vi "Read Variable (integer).vi"(8 "error in (no error)":errorcluster, 9 "Datatype":i32, 10 "PG path":string, 11 "Data.PGQL in":refnum<class "LV-Data.PGSQL.lvclass">) -> (0 "error out":errorcluster, 1 "Time Stamp":timestamp=timestamp(-9593186400 s since 1904-01-01), 2 "Value":i32, 3 "Data.PGSQL out":refnum<class "LV-Data.PGSQL.lvclass">, 4 "Column (units)":string, 5 "SQL string":string)   [LabVIEW 2019, in "LV-Data.PGSQL.lvclass"]
uses:
  LV-Data.PGSQL.lvclass
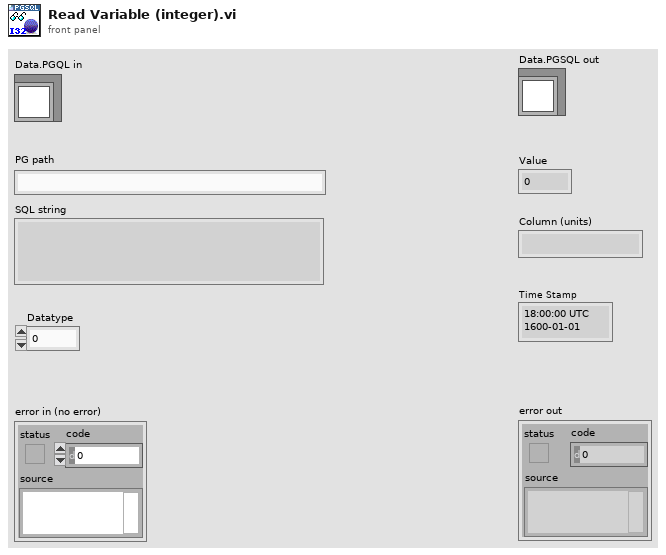
[diagram p1: front panel]
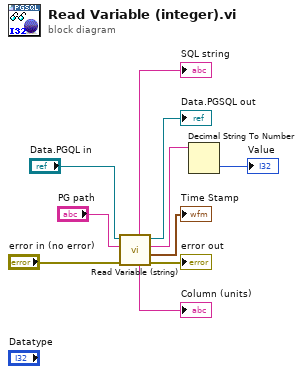
[diagram p0: block diagram]
diagram:
  n1 = call "Read Variable (string).vi"("error in (no error)"="error in (no error)", "PG path"="PG path", "Data.PGQL in"="Data.PGQL in") -> ("error out"=→"error out":errorcluster, "Time Stamp"=→"Time Stamp":timestamp, "Value"=w5:string, "Data.PGSQL out"=→"Data.PGSQL out":refnum<class "LV-Data.PGSQL.lvclass">, "Column (units)"=→"Column (units)":string, "SQL string"=→"SQL string":string)  [unwired: 3 in]
  n2 = Decimal String To Number(string=w5) -> (number=→"Value":i32)  [unwired: 2 in, 1 out]
